vi "RaiseElevator.vi"() -> ()   [LabVIEW 2018]
uses:
  Framework/Robot Global Data.vi
panel:
  in  "NoWait":bool
  in  "Height":dbl
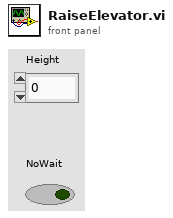
[diagram p1: front panel]
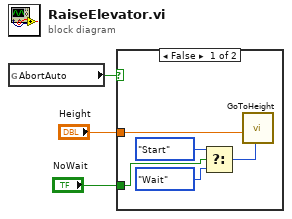
[diagram p0: block diagram]
diagram:
  n1 = global read "Robot Global Data.vi" "AbortAuto"() -> (w3:bool)
  n2 = case shown="False" w3 {
    tunnel: "NoWait" -> [w6 _]
    tunnel: "Height" -> [w5 _]
    frame False {
      n3 = Select(t=enum16{"Start", "Wait"}."Start", s=w6, f=enum16{"Start", "Wait"}."Wait" ("Synchronication")) -> (s? t:f=w4:enum16{"Start", "Wait"})
      n4 = call "GoToHeight.vi"("Synchronization"=w4, "Setpoint"=w5) -> ()  [unwired: 9 in, 1 out]
    }
    frame True {
    }
  }
